vi "PerfAddRemove.vi"() -> (3 "Add time":dbl format="%.2p")   [LabVIEW 2024, in "RefTypedCircularBuffer.Tests.Perf.lvlib"]
uses:
  RefTypedCircularBuffer.Tests.Perf.lvlib
  Type.ctl
  RefTypedCircularBuffer.lvclass/RefTypedCircularBuffer.ctl
  <vilib>/Analysis/baseanly.llb/Mean (DBL).vi
  <vilib>/Analysis/NI_AALBase.lvlib
  RefTypedCircularBuffer.lvclass
panel:
  out "remove time":dbl format="%.2p"
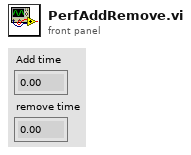
[diagram p1: front panel]
types:
  T1 = typedef "RefTypedCircularBuffer.lvclass/Type.ctl" = u8
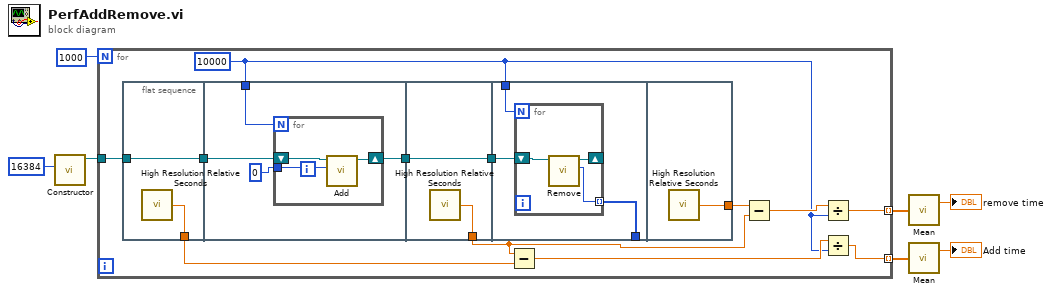
[diagram p0: block diagram]
diagram:
  n1 = call "Constructor.vi"("Capacity"=u32 16384) -> ("TypedCircularBuffer out"=w2:refnum<class "RefTypedCircularBuffer.lvclass">)  [unwired: 10 in]
  n2 = for {
    N: 1000 -> [_]
    tunnel: [w11] -> w7 mode=indexing
    tunnel: w2 -> [w18]
    tunnel: [w8] -> w3 mode=indexing
    w9 = 10000
    n3 = flat-sequence {
      tunnel: w18 -> [w21]
      tunnel: [w21] -> w15
      tunnel: [w20] -> w13
      tunnel: [w24] -> w16
      tunnel: w15 -> [w25]
      tunnel: w9 -> [w23]
      tunnel: [w30] -> w14
      tunnel: [w29] -> w17
      tunnel: w16 -> [w29]
      tunnel: [w33] -> _
      tunnel: w17 -> [w32]
      tunnel: w9 -> [w31]
      tunnel: [w37] -> w19
      frame #0 {
        n4 = call <vilib>:"High Resolution Relative Seconds.vi"() -> ("relative seconds"=w20:dbl)
      }
      frame #1 {
        n5 = for {
          N: w23 -> [_]
          shift-right: [w27] -> w24
          shift-left: w25 -> [w28]
          tunnel: T1 0 ("Element") -> [w26]
          n6 = call "Add.vi"("Element"=w26, "TypedCircularBuffer in"=w28) -> ("TypedCircularBuffer out"=w27:refnum<class "RefTypedCircularBuffer.lvclass">)  [unwired: 7 in, 2 out]
        }
      }
      frame #2 {
        n7 = call <vilib>:"High Resolution Relative Seconds.vi"() -> ("relative seconds"=w30:dbl)
      }
      frame #3 {
        n8 = for {
          N: w31 -> [_]
          shift-right: [w35] -> _
          shift-left: w32 -> [w36]
          tunnel: [w34] -> w33 mode=indexing
          n9 = call "Remove.vi"("TypedCircularBuffer in"=w36) -> ("element"=w34:T1, "TypedCircularBuffer out"=w35:refnum<class "RefTypedCircularBuffer.lvclass">)  [unwired: 8 in, 1 out]
        }
      }
      frame #4 {
        n10 = call <vilib>:"High Resolution Relative Seconds.vi"() -> ("relative seconds"=w37:dbl)
      }
    }
    n11 = Subtract(x=w14, y=w13) -> (x-y=w10:dbl)
    n12 = Subtract(x=w19, y=w14) -> (x-y=w12:dbl)
    n13 = Divide(x=w12, y=w9) -> (x/y=w11:dbl)
    n14 = Divide(x=w10, y=w9) -> (x/y=w8:dbl)
  }
  n15 = call-poly <vilib>:"Mean.vi"("X"=w7) -> ("mean"=→"remove time":dbl)  [unwired: 1 out]
  n16 = call-poly <vilib>:"Mean.vi"("X"=w3) -> ("mean"=→"Add time":dbl)  [unwired: 1 out]
